vi "Table, Set Row Labels, Numeric.vi"(8 "error in":errorcluster, 9 "step (1)":i32=1, 10 "start (0)":i32, 11 "Tbl Refnum":refnum<vi>) -> (0 "error out":errorcluster, 3 "Tbl Refnum out":refnum<vi>)   [LabVIEW 2010]
doc: "Sequentially numbers the table row labels (headers). Existing table row labels will be deleted."
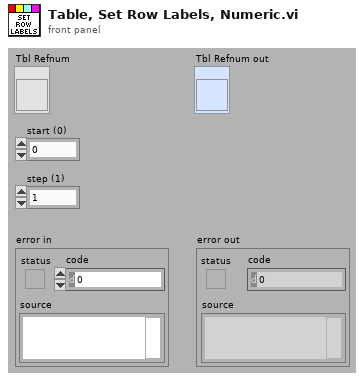
[diagram p1: front panel]
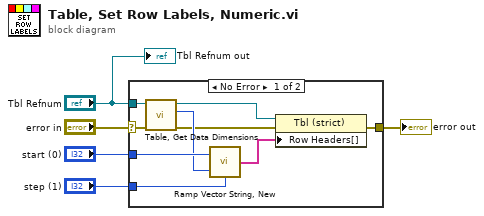
[diagram p0: block diagram]
diagram:
  n1 = case shown="No Error" "error in" {
    selector: "error in" -> [w6 w15]
    tunnel: "step (1)" -> [w13 _]
    tunnel: "start (0)" -> [w12 _]
    tunnel: [w11 w15] -> w3
    tunnel: "Tbl Refnum" -> [w7 _]
    frame No Error {
      n2 = call "Table, Get Data Dimensions.vi"("error in"=w6, "Tbl Refnum"=w7) -> ("error out"=w9:errorcluster, "row_n"=w10:i32, "Tbl Refnum out"=w8:refnum<vi>)  [unwired: 6 in, 1 out]
      n3 = call "Ramp Vector String, New.vi"("step (1)"=w13, "nelem"=w10, "start (0)"=w12) -> ("ramp"=w14:string[])
      n4 = property class="Tbl (strict)"(reference=w8, error in=w9, "Row Headers[]"=w14) -> (error out=w11:errorcluster)  [unwired: 1 out]
    }
    frame Error {
    }
  }
  "error out" <- w3
  "Tbl Refnum out" <- "Tbl Refnum"
